vi "Test ID Encode.vi"() -> ()   [LabVIEW 2021]
uses:
  typedef/ISO FD Frame Type.ctl
  CAN_Logic.lvclass
panel:
  out "ISO FD Type out":T1
  out "Extended ID out":bool
  out "Frame ID out":u32
  in  "Extended ID":bool
  in  "Frame ID in":u32=12
  in  "ISO FD Type":T1
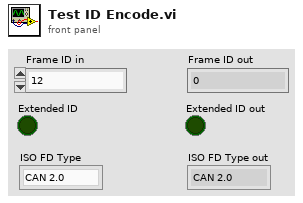
[diagram p1: front panel]
types:
  T1 = typedef "CAN_Logic.lvclass/ISO FD Frame Type.ctl" = enum16{"CAN 2.0", "FD", "FD+BRS"}
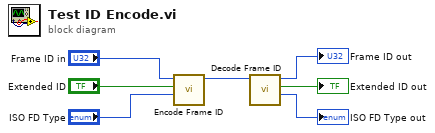
[diagram p0: block diagram]
diagram:
  n1 = call "Encode Frame ID.vi"("ISO FD Type"="ISO FD Type", "Extended ID"="Extended ID", "Frame ID in"="Frame ID in") -> ("Frame ID out"=w7:u32)  [unwired: 8 in]
  n2 = call "Decode Frame ID.vi"("Frame ID in"=w7) -> ("ISO FD Type"=→"ISO FD Type out":T1, "Extended ID"=→"Extended ID out":bool, "Frame ID out"=→"Frame ID out":u32)  [unwired: 8 in]
